vi "check.vi"(9 "Password":string caption="密   码:", 11 "UserName":string caption="用户名:") -> (0 "管理员":bool, 2 "Success?":bool)   [LabVIEW 2020]
uses:
  <vilib>/Utility/file.llb/Read Delimited Spreadsheet (string).vi
  <userlib>/_OpenG.lib/array/array.llb/Search 1D Array (String)__ogtk.vi
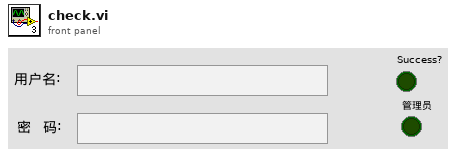
[diagram p1: front panel]
types:
  T1 = enum16{"open", "replace", "create", "open or create", "replace or create", "replace or create with confirmation"}
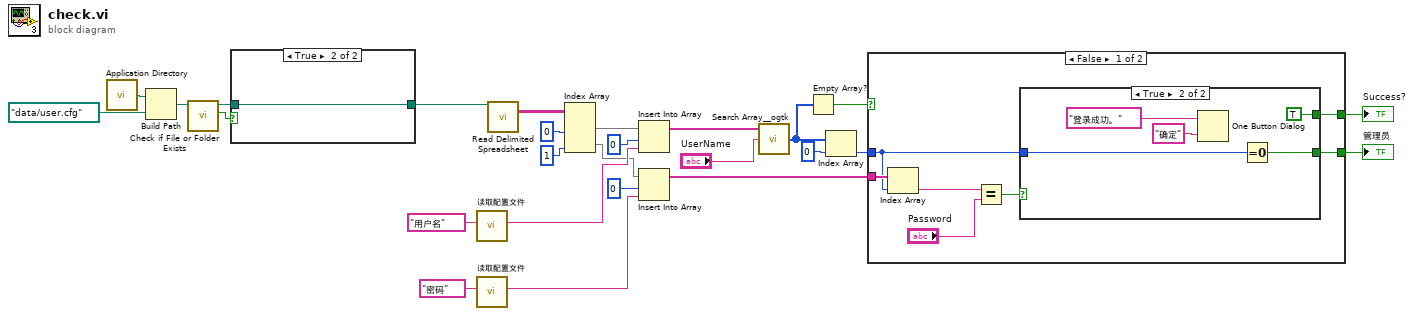
[diagram p0: block diagram]
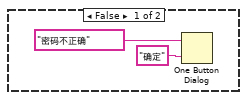
[diagram p2: hidden frame]
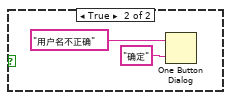
[diagram p3: hidden frame]
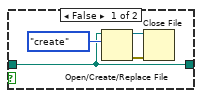
[diagram p4: hidden frame]
diagram:
  n1 = call <vilib>:"Application Directory.vi"() -> ("Application Directory"=w22:path)
  n2 = Build Path(base path=w22, name or relative path=path "data/user.cfg") -> (appended path=w23:path)
  n3 = call <vilib>:"Check if File or Folder Exists.vi"("path"=w23) -> ("file or folder exists?"=w24:bool, "dup path"=w25:path)  [unwired: 8 in, 1 out]
  n4 = case shown="True" w24 {
    tunnel: w25 -> [w27 w31]
    tunnel: [w27 w31] -> w26
    frame False {
      n5 = Open/Create/Replace File(file path (use dialog)=w27, operation (0:open)=T1."create" ("操作(0:open)")) -> (refnum out=w28:refnum<file>, error out=w29:errorcluster)  [unwired: 4 in, 1 out]
      n6 = Close File(refnum=w28, error in=w29) -> ()  [unwired: 2 out]
    }
    frame True {
    }
  }
  n7 = call "读取配置文件.vi"("配置"="用户名") -> ("路径"=w11:string)  [unwired: 9 in, 1 out]
  n8 = call "读取配置文件.vi"("配置"="密码") -> ("路径"=w7:string)  [unwired: 9 in, 1 out]
  n9 = call-poly <vilib>:"Read Delimited Spreadsheet.vi"("file path (dialog if empty)"=w26) -> ("all rows"=w20:string[][])  [unwired: 9 in, 5 out]
  n10 = Index Array(array=w20, index (col) #1=0 ("禁用的索引 (列)"), index (col) #2=1 ("禁用的索引 (列)")) -> (element #1=w12:string[], element #2=w6:string[])  [unwired: 2 in]
  n11 = Insert Into Array(array=w12, index=0 ("索引"), new element=w11) -> (w5:string[])
  n12 = Insert Into Array(array=w6, index=0 ("索引"), new element=w7) -> (w4:string[])
  n13 = call-poly <userlib>:"Search Array__ogtk.vi"("Array"=w5, "Element Data"="UserName") -> ("Indices of Elements"=w16:i32[])  [unwired: 7 in]
  n14 = Empty Array?(array=w16) -> (empty?=w15:bool)
  n15 = Index Array(array=w16, index=0 ("索引")) -> (element=w14:i32)
  n16 = case shown="False" w15 {
    tunnel: w4 -> [w38 _]
    tunnel: w14 -> [w34 _]
    tunnel: [w35 _] -> w3
    tunnel: [w33 _] -> w2
    frame False {
      n17 = Index Array(array=w38, index=w34) -> (element=w37:string)
      n18 = Equal?(x=w37, y="Password") -> (x = y?=w36:bool)
      n19 = case shown="True" w36 {
        tunnel: [_ TRUE] -> w35
        tunnel: w34 -> [_ w42]
        tunnel: [_ w41] -> w33
        frame False {
          n20 = One Button Dialog(message="密码不正确", button name ("OK")="确定") -> ()  [unwired: 1 out]
        }
        frame True {
          n21 = One Button Dialog(message="登录成功。", button name ("OK")="确定") -> ()  [unwired: 1 out]
          n22 = Equal To 0?(x=w42) -> (x = 0?=w41:bool)
        }
      }
    }
    frame True {
      n23 = One Button Dialog(message="用户名不正确", button name ("OK")="确定") -> ()  [unwired: 1 out]
    }
  }
  "Success?" <- w3
  "管理员" <- w2
